vi "readStatusNotifier.vi"(8 "error in (no error)":errorcluster, 9 "notification in":bool, 10 "serverSelection":enum16{"cmd", "tel"}(ring), 11 "TcpServer in":refnum<class "TcpServer.lvclass">) -> (0 "error out (no error)":errorcluster, 1 "notification out":bool, 3 "TcpServer out":refnum<class "TcpServer.lvclass">)   [LabVIEW 2018, in "TcpServer.lvclass"]
doc: "Read the Status Notifier from tcpServerStateMachine.vi.\n\nNote: Put this VI in Prealocated reentrant clone execution."
uses:
  TcpServer.lvclass
  TcpServer.lvclass/TcpServer.ctl
  TcpServerBase/TcpServerBase.lvclass/TcpServerBase.ctl
  TcpServerCmd/TcpServerCmd.lvclass
  home/pcortes/github/ts_labview_tcp_json/src/TcpServerBase/TcpServerBase.lvclass
  TcpServerTel/TcpServerTel.lvclass
  TcpServerBase/TcpServerBase.lvclass
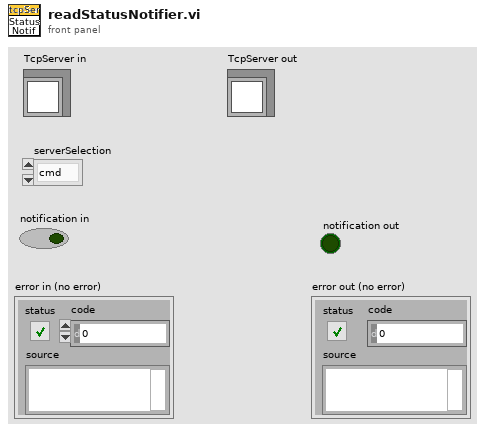
[diagram p1: front panel]
types:
  T1 = cluster{"connectionStatus":bool, "errorSource":string}
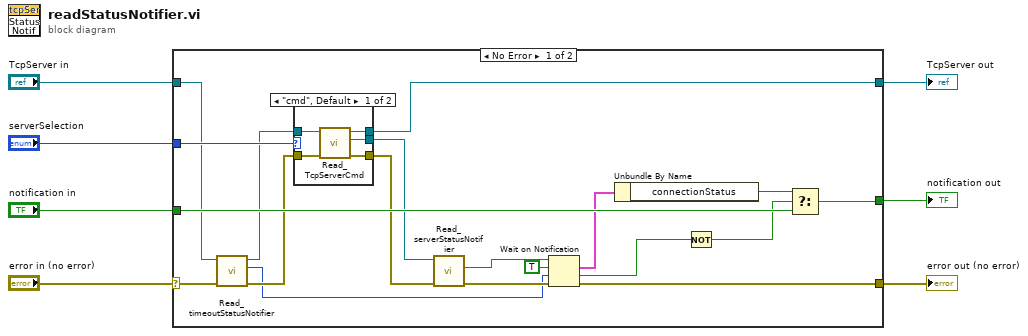
[diagram p0: block diagram]
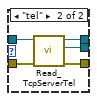
[diagram p2: hidden frame]
diagram:
  n1 = case shown="No Error" "error in (no error)" {
    selector: "error in (no error)" -> [w12 w38]
    tunnel: [w26 w39] -> w7
    tunnel: "notification in" -> [w24 w39]
    tunnel: [w17 w38] -> w4
    tunnel: [w16 w37] -> w2
    tunnel: "TcpServer in" -> [w11 w37]
    tunnel: "serverSelection" -> [w15 _]
    frame No Error {
      n2 = call "Read_timeoutStatusNotifier.vi"("error in (no error)"=w12, "TcpServer in"=w11) -> ("error out"=w10:errorcluster, "timeoutStatusNotifier"=w8:i32, "TcpServer out"=w9:refnum<class "TcpServer.lvclass">)  [unwired: 7 in]
      n3 = case shown="\"cmd\", Default" w15 {
        tunnel: [w31 w36] -> w16
        tunnel: [w30 w34] -> w14
        tunnel: [w29 w35] -> w13
        tunnel: w10 -> [w27 w33]
        tunnel: w9 -> [w28 w32]
        frame "cmd", Default {
          n4 = call "Read_TcpServerCmd.vi"("error in (no error)"=w27, "TcpServer in"=w28) -> ("error out"=w29:errorcluster, "TcpServerCmd.lvclass"=w30:refnum<class "TcpServerCmd.lvclass">, "TcpServer out"=w31:refnum<class "TcpServer.lvclass">)  [unwired: 7 in]
        }
        frame "tel" {
          n5 = call "Read_TcpServerTel.vi"("error in (no error)"=w33, "TcpServer in"=w32) -> ("error out"=w35:errorcluster, "TcpServerTel.lvclass"=w34:refnum<class "TcpServerTel.lvclass">, "TcpServer out"=w36:refnum<class "TcpServer.lvclass">)  [unwired: 7 in]
        }
      }
      n6 = call "Read_serverStatusNotifier.vi"("error in (no error)"=w13, "TcpServerBase in"=w14) -> ("error out"=w23:errorcluster, "serverStatusNotifier"=w19:refnum<notifier>)  [unwired: 7 in, 1 out]
      n7 = Wait on Notification(notifier=w19, ignore previous (F)=TRUE, timeout in ms (-1)=w8, error in (no error)=w23) -> (notification=w18:T1, timed out?=w22:bool, error out=w17:errorcluster)  [unwired: 1 out]
      n8 = Unbundle By Name(w18) -> ("connectionStatus"=w25:bool)
      n9 = Not(x=w22) -> (.not. x?=w21:bool)
      n10 = Select(t=w25, s=w21, f=w24) -> (s? t:f=w26:bool)
    }
    frame Error {
    }
  }
  "notification out" <- w7
  "error out (no error)" <- w4
  "TcpServer out" <- w2
